vi "MES.VI"   [LabVIEW 2018]
uses:
  MentorAPI.dll
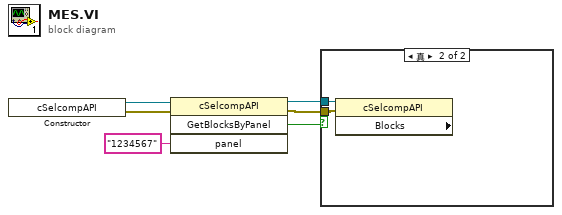
[diagram p0: block diagram]
diagram:
  n1 = constructor class="cSelcompAPI"() -> (reference out=w3:refnum<k24>, error out=w2:errorcluster)  [unwired: 3 in, 1 out]
  n2 = invoke class="cSelcompAPI" method="GetBlocksByPanel"(reference=w3, error in=w2, "panel"="1234567") -> (reference out=w5:refnum<k24>, error out=w4:errorcluster, "GetBlocksByPanel"=w6:bool)  [unwired: 1 in, 1 out]
  n3 = case shown="真" w6 {
    tunnel: w5 -> [_ w8]
    tunnel: w4 -> [_ w7]
    frame False {
    }
    frame True {
      n4 = property class="cSelcompAPI" props=["Blocks"](reference=w8, error in=w7) -> ()  [unwired: 3 out]
    }
  }
